vi "Capture2D.vi"(0 "Camera Reference in":refnum<k24>, 1 "error in":errorcluster) -> (2 "Camera Reference out":refnum<k24>, 3 "error out":errorcluster, 4 "GrayScaleImage Reference out":refnum<k24>, 5 "Color2DImage Reference out":refnum<k24>)   [LabVIEW 2023]
uses:
  C:/Mech-Mind/Mech-Eye SDK-2.5.0-b5-dev-01-03/API/dll/net48/MechEyeApiNet.dll
  dll/net48/MechEyeApiNet.dll
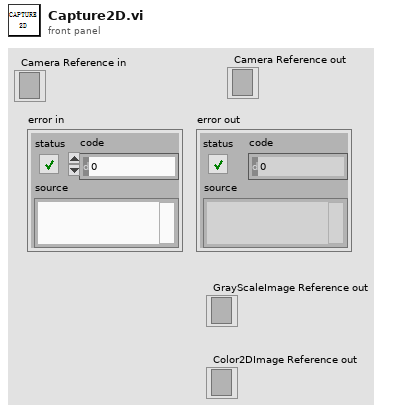
[diagram p1: front panel]
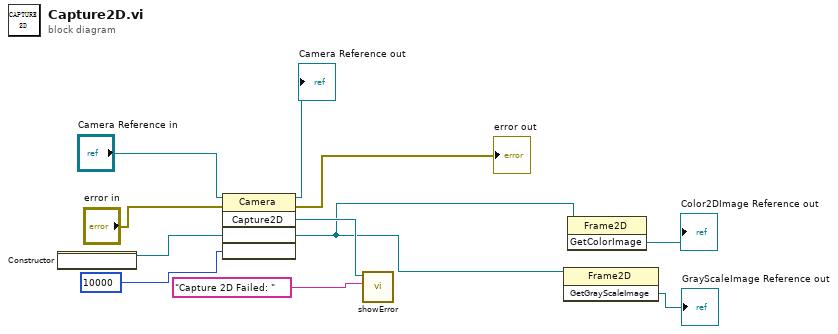
[diagram p0: block diagram]
diagram:
  n1 = constructor class="Frame2D"() -> (reference out=w10:refnum<k24>)  [unwired: 3 in, 2 out]
  n2 = invoke on="Invoke Node" class="Camera" method="Capture2D"(reference="Camera Reference in", error in="error in", w10, 10000) -> (reference out=→"Camera Reference out":refnum<k24>, error out=→"error out":errorcluster, w8:refnum<k24>, w5:refnum<k24>)  [unwired: 1 in, 1 out]
  n3 = call "showError.vi"(10:"Capture 2D Failed: ", 11:w8) -> ()  [unwired: 10 in]
  n4 = invoke class="Frame2D" method="GetGrayScaleImage"(reference=w5) -> (→"GrayScaleImage Reference out":refnum<k24>)  [unwired: 2 in, 2 out]
  n5 = invoke class="Frame2D" method="GetColorImage"(reference=w5) -> (→"Color2DImage Reference out":refnum<k24>)  [unwired: 2 in, 2 out]
